vi "Move Waveform in List.vi"(8 "error in (no error)":errorcluster, 9 "After Move Index":i32, 10 "Before Move Index":i32, 11 "Canvas Wfm Array In":waveform(dbl)[](array[waveform])) -> (0 "error out":errorcluster, 3 "Canvas Wfm Array Out":waveform(dbl)[](array[waveform]))   [LabVIEW 2025, in "TDMS Waveform Creator UI.lvlib"]
uses:
  TDMS Waveform Creator UI.lvlib
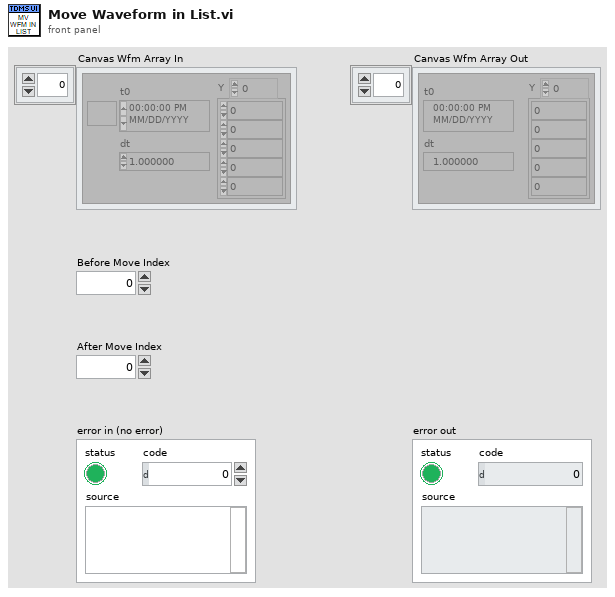
[diagram p1: front panel]
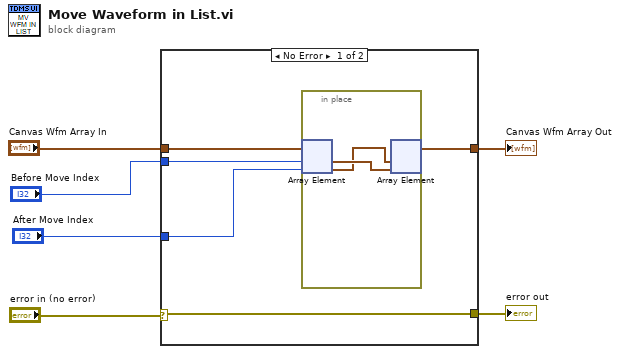
[diagram p0: block diagram]
diagram:
  n1 = case shown="No Error" "error in (no error)" {
    selector: "error in (no error)" -> [w7 w15]
    tunnel: "Canvas Wfm Array In" -> [w11 w14]
    tunnel: [w10 w14] -> w4
    tunnel: [w7 w15] -> w3
    tunnel: "Before Move Index" -> [w9 _]
    tunnel: "After Move Index" -> [w8 _]
    frame No Error {
      n2 = in-place {
        n3 = in-place-array #1(w11, w9, w8) -> (w13:waveform(dbl), w12:waveform(dbl))
        n4 = in-place-array #1(w12, w13) -> (w10:waveform(dbl)[])  [unwired: 2 out]
      }
    }
    frame Error {
    }
  }
  "error out" <- w3
  "Canvas Wfm Array Out" <- w4
